vi "GetRxSynthBands.vi"(8 "error in (no error)":errorcluster) -> (0 "error out":errorcluster, 2 "SynthBands":T1(array[cluster]))   [LabVIEW 2011]
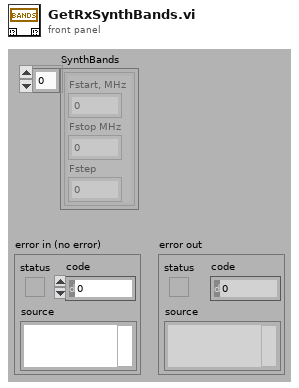
[diagram p1: front panel]
types:
  T1 = cluster{"Fstart, MHz":dbl, "Fstop MHz":dbl, "Fstep":dbl}[]
  T2 = cluster{"Fstart":dbl, "Fstop":dbl, "SyStep":dbl}[]
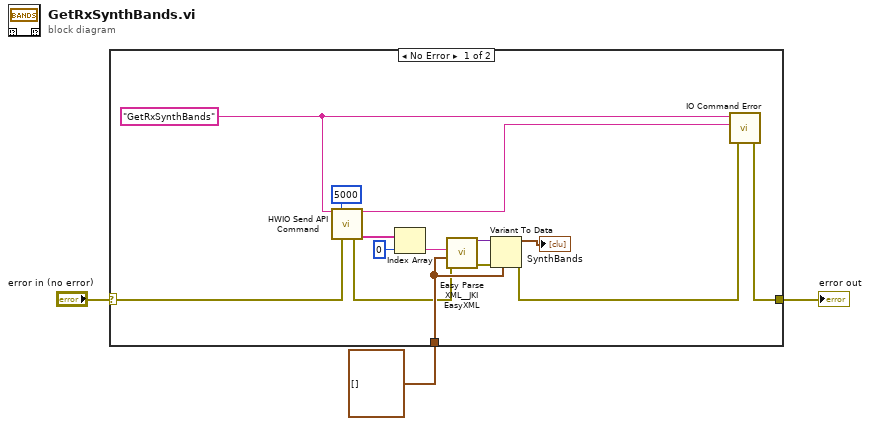
[diagram p0: block diagram]
diagram:
  n1 = case shown="No Error" "error in (no error)" {
    selector: "error in (no error)" -> [w14 w18]
    tunnel: [w15 w18] -> w3
    tunnel: T2 [] ("SYBands") -> [w12 _]
    frame No Error {
      w17 = "GetRxSynthBands"
      n2 = call "HWIO Send API Command.vi"("Action"=w17, "Timeout ms (5000)"=5000 ("PerCommand Timeout (ms)"), "error in (no error)"=w14) -> ("Action out"=w16:string, "error out"=w5:errorcluster, "String out"=w11:string[])  [unwired: 5 in, 5 out]
      n3 = Index Array(array=w11, index=0) -> (element=w9:string)
      n4 = call "Easy Parse XML__JKI EasyXML.vi"("error in (no error)"=w5, "LabVIEW Data (Type)"=w12, "XML String"=w9) -> ("error out"=w6:errorcluster, "LabVIEW Data"=w8:variant)  [unwired: 7 in]
      n5 = Variant To Data(error in=w6, type=w12, Variant=w8) -> (data=→"SynthBands":T2, error out=w4:errorcluster)
      n6 = call "IO Command Error.vi"("error in (no error)"=w4, "Command Returned (\"\")"=w16, "Command Sent (\"\")"=w17) -> ("error out"=w15:errorcluster)  [unwired: 4 out]
    }
    frame Error {
    }
  }
  "error out" <- w3
